vi "get_temp_folder_path.vi"(8 "error in (no error)":errorcluster, 10 "flush?":bool, 11 "GenericComponent in":refnum<class "GenericComponent.lvclass">) -> (0 "error out":errorcluster, 2 "temp path":path, 3 "GenericComponent out":refnum<class "GenericComponent.lvclass">)   [LabVIEW 2010, in "GenericComponent.lvclass"]
uses:
  GenericComponent.lvclass
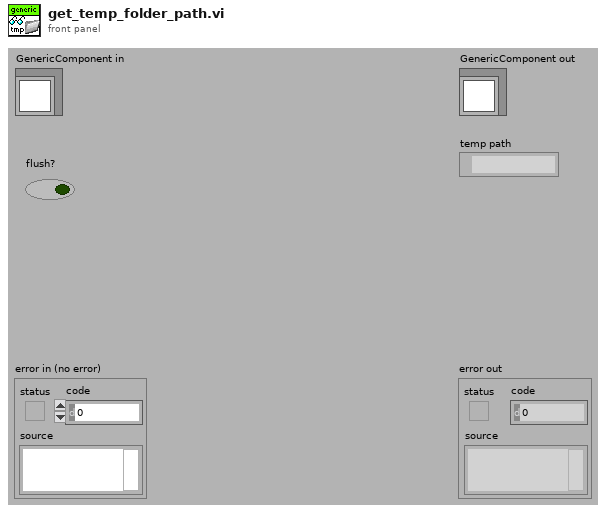
[diagram p1: front panel]
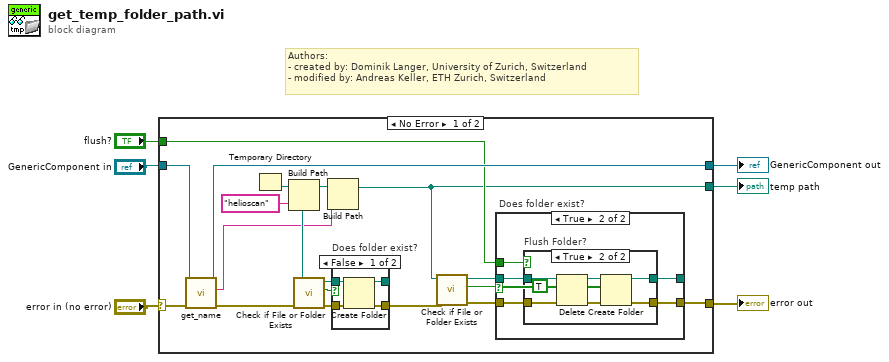
[diagram p0: block diagram]
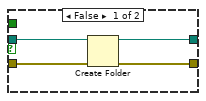
[diagram p2: hidden frame]
diagram:
  # "Authors: \n- created by: Dominik Langer, University of Zurich, Switzerland\n- modified by: Andreas Keller, ETH Zurich, Switzerland"
  n1 = case shown="No Error" "error in (no error)" {
    selector: "error in (no error)" -> [w20 w50]
    tunnel: [w11 w50] -> w5
    tunnel: [w21 w49] -> w3
    tunnel: "GenericComponent in" -> [w22 w49]
    tunnel: [w8 _] -> w2
    tunnel: "flush?" -> [w10 _]
    frame No Error {
      n2 = call-dynamic "get_name.vi"("error in (no error)"=w20, "GenericPlugin in"=w22) -> ("error out"=w16:errorcluster, "component name"=w7:string, "GenericPlugin out"=w21:refnum<class "GenericComponent.lvclass">)  [unwired: 7 in]
      n3 = Temporary Directory() -> (w23:path)
      n4 = Build Path(base path=w23, name or relative path="helioscan") -> (appended path=w9:path)
      n5 = call <vilib>:"Check if File or Folder Exists.vi"("error in (no error)"=w16, "path"=w9) -> ("error out"=w18:errorcluster, "file or folder exists?"=w17:bool, "dup path"=w19:path)  [unwired: 7 in]
      n6 = Build Path(base path=w9, name or relative path=w7) -> (appended path=w8:path)
      n7 = case "Does folder exist?" shown="False" w17 {
        tunnel: w19 -> [w46 w47]
        tunnel: w18 -> [w45 w48]
        tunnel: [w44 w48] -> w12
        tunnel: [w43 w47] -> _
        frame False {
          n8 = Create Folder(path (use dialog)=w46, error in=w45) -> (created path=w43:path, error out=w44:errorcluster)  [unwired: 1 in, 1 out]
        }
        frame True {
        }
      }
      n9 = call <vilib>:"Check if File or Folder Exists.vi"("error in (no error)"=w12, "path"=w8) -> ("error out"=w14:errorcluster, "file or folder exists?"=w13:bool, "dup path"=w15:path)  [unwired: 7 in]
      n10 = case "Does folder exist?" shown="True" w13 {
        tunnel: w15 -> [w26 w32]
        tunnel: w14 -> [w25 w33]
        tunnel: [w28 w30] -> w11
        tunnel: [w27 w31] -> _
        tunnel: w10 -> [_ w29]
        frame False {
          n11 = Create Folder(path (use dialog)=w26, error in=w25) -> (created path=w27:path, error out=w28:errorcluster)  [unwired: 1 in, 1 out]
        }
        frame True {
          n12 = case "Flush Folder?" shown="True" w29 {
            tunnel: w32 -> [w35 w42]
            tunnel: w33 -> [w34 w37]
            tunnel: [w35 w39] -> w31
            tunnel: [w34 w38] -> w30
            frame False {
            }
            frame True {
              n13 = Delete(path (use dialog)=w42, entire hierarchy (F)=TRUE, error in=w37) -> (deleted path=w41:path, error out=w40:errorcluster)  [unwired: 2 in, 1 out]
              n14 = Create Folder(path (use dialog)=w41, error in=w40) -> (created path=w39:path, error out=w38:errorcluster)  [unwired: 1 in, 1 out]
            }
          }
        }
      }
    }
    frame Error {
    }
  }
  "error out" <- w5
  "GenericComponent out" <- w3
  "temp path" <- w2
